vi "UHR-Fleezers Control (host) -TL FB Corrected Ronen semipassive - stepping.vi"(0 "Tab Control":T5(tab)=enum."Trap Control (RF)") -> ()   [LabVIEW 2013] (continued)
                      n1354 = To Double Precision Float(number=w2139) -> (double precision float=w2138:cluster{"Horizontal":dbl, "Vertical":dbl})
                      n1355 = Multiply(x=cluster{"Horizontal":dbl, "Vertical":dbl} {"Horizontal"=-1.0, "Vertical"=1.0}, y="Manipulation Scaling") -> (x*y=w2134:cluster{"Horizontal":dbl, "Vertical":dbl})
                      n1356 = local read "X RF Frequency Limits (MHz)"() -> (w2100:T17)
                      n1357 = Multiply(x=w2138, y=w2134) -> (x*y=w2136:cluster{"Horizontal":dbl, "Vertical":dbl})
                      n1358 = Unbundle By Name(w2136) -> ("Horizontal"=w2131:dbl, "Vertical"=w2135:dbl)
                      n1359 = Unbundle By Name(w2099) -> ("Maximum"=w2102:dbl, "Minimum"=w2101:dbl)
                      n1360 = Boolean To (0,1)(Boolean="Manip. X?") -> (0, 1=w2129:i16)
                      n1361 = Boolean To (0,1)(Boolean="Manip. Y?") -> (0, 1=w2126:i16)
                      n1362 = local read "BD 1 Frequency 2 (MHz)"() -> (w2116:dbl)
                      n1363 = Multiply(x=w2135, y=w2126) -> (x*y=w2128:dbl)
                      n1364 = Multiply(x=w2129, y=w2131) -> (x*y=w2132:dbl)
                      n1365 = local read "BD 2 Frequency 2 (MHz)"() -> (w2115:dbl)
                      n1366 = Unbundle By Name(w2100) -> ("Maximum"=w2104:dbl, "Minimum"=w2103:dbl)
                      n1367 = Add(x=w2113, y=w2128) -> (x+y=w2106:dbl)
                      n1368 = Add(x=w2114, y=w2132) -> (x+y=w2108:dbl)
                      n1369 = In Range and Coerce(upper limit=w2104, x=w2108, lower limit=w2103) -> (coerced(x)=w2107:dbl)  [unwired: 1 out]
                      n1370 = In Range and Coerce(upper limit=w2102, x=w2106, lower limit=w2101) -> (coerced(x)=w2105:dbl)  [unwired: 1 out]
                      n1371 = Subtract(x=w2107, y=w2116) -> (x-y=w2125:dbl)
                      n1372 = Subtract(x=w2105, y=w2115) -> (x-y=w2124:dbl)
                      n1373 = Square(x=w2125) -> (x^2=w2123:dbl)
                      n1374 = Square(x=w2124) -> (x^2=w2122:dbl)
                      n1375 = Add(x=w2123, y=w2122) -> (x+y=w2121:dbl)
                      n1376 = Square Root(x=w2121) -> (sqrt(x)=w2117:dbl)
                      n1377 = In Range and Coerce(upper limit="Limit Max (MHz)", x=w2117, lower limit="Limit Min (MHz)") -> (In Range?=w2110:bool)  [unwired: 1 out]
                      n1378 = Not(x="Limits Enable") -> (.not. x?=w2109:bool)
                      n1379 = Or(x=w2110, y=w2109) -> (x .or. y?=w2111:bool)
                      n1380 = case shown="True" w2111 {
                        tunnel: w2118 -> [_ w2151]
                        tunnel: w2117 -> [_ w2142]
                        tunnel: w2107 -> [_ w2149]
                        tunnel: w2116 -> [_ w2148]
                        tunnel: w2105 -> [_ w2147]
                        tunnel: w2115 -> [_ w2146]
                        tunnel: w2100 -> [_ w2144]
                        tunnel: w2099 -> [_ w2143]
                        frame False {
                        }
                        frame True {
                          n1381 = local read "BD 1 Frequency 3 (MHz)"() -> (w2150:dbl)
                          n1382 = local read "BD 2 Frequency 3 (MHz)"() -> (w2145:dbl)
                          n1383 = local write "Trap Delta (MHz)"(w2142) -> ()
                          n1384 = property on="Initial delta (MHz)" class="DigNum (strict)"("Val(Sgnl)"=w2142) -> ()  [unwired: 2 in, 2 out]
                          n1385 = call "set RF board frequency - interlace.vi"("Board 2 Frequency Limits"=w2143, "Board 1 Frequency Limits"=w2144, "FPGA VI Reference In"=w2151, "Board 2 Frequency 3 (MHz)"=w2145, "Board 1 Frequency 3 (MHz)"=w2150, "Board 2 Frequency 2 (MHz)"=w2146, "Board 2 Frequency 1 (MHz)"=w2147, "Board 1 Frequency 2 (MHz)"=w2148, "Board 1 Frequency 1  (MHz)"=w2149) -> ()  [unwired: 1 in, 2 out]
                          n1386 = local write "BD 2 Frequency 1 (MHz)"(w2147) -> ()
                          n1387 = local write "BD 1 Frequency 1 (MHz)"(w2149) -> ()
                        }
                      }
                    }
                    frame True {
                    }
                  }
                }
                event Mouse Up {
                  n1388 = event-data() -> ("Button"=w2152:u16)  [unwired: 8 out]
                  n1389 = case shown="3" w2152 {
                    tunnel: [FALSE TRUE] -> w2153
                    frame 0, Default {
                    }
                    frame 3 {
                      n1390 = local write "Manipulating Trap"(FALSE ("Manipulating Trap")) -> ()
                    }
                  }
                }
              }
            }
          }
        }
      }
      event Mouse Move {
        n1391 = event-data() -> ()  [unwired: 6 out]
      }
    }
    n1392 = local read "Stop All"() -> (w1974:bool)
    n1393 = node-c288() -> ()  [unwired: 2 out]
  }
  n1394 = node-c288(w34) -> ()  [unwired: 1 out]
  n1395 = node-c288(w88) -> ()  [unwired: 1 out]
  n1396 = node-c288(w95) -> ()  [unwired: 1 out]
  n1397 = node-c288(i64 1 ("Period"), 1 ("Processor")) -> (w182:T25)  [unwired: 2 out]
  n1398 = timed-loop "Acquire Data" {
    tunnel: w44 -> [w2440]
    tunnel: w60 -> [w2439]
    tunnel: [w2470] -> w53
    tunnel: [w2464] -> w52
    timing: w182 -> [_]
    timing-out: [_] -> w181
    tunnel: w79 -> [w2276]
    stop <- "Stop All" stop-if-true
    (unwired) u32 0 ("Number of Elements")
    w2263 = "NI_ChannelName" ("name")
    n1399 = node-c288() -> ()  [unwired: 2 out]
    n1400 = First Call?() -> (First Call?: T/F=w2229:bool)
    n1401 = Or(x="Reset", y=w2229) -> (x .or. y?=w2230:bool)
    n1402 = local read "MCL Tracking"() -> (w2167:bool)
    n1403 = case "Reset data stream" shown="True" w2230 {
      tunnel: w2440 -> [w2582 w2590]
      tunnel: w2439 -> [w2581 w2589]
      tunnel: [w2582 w2584] -> w2165
      tunnel: [w2581 w2583] -> w2435
      frame False {
      }
      frame True {
        w2587 = TRUE ("AI to FIFO")
        n1404 = local write "Overflow (data lost)"(FALSE ("Overflow (data lost)")) -> ()
        n1405 = call "reset FPGA DMA.vi"("error in"=w2589, "FPGA VI Reference In"=w2590) -> ("error out"=w2585:errorcluster, "FPGA VI Reference Out"=w2586:T20)
        n1406 = xnode "Read/Write Control"("FPGA VI Reference In"=w2586, "error in"=w2585, "AI to FIFO"=w2587, "APD to FIFO"=w2587) -> ("FPGA VI Reference Out"=w2584:T20, "error out"=w2583:errorcluster)
      }
    }
    n1407 = Or(x="Start AOD Scan", y="Trap Raster Scan") -> (x .or. y?=w2391:bool)
    n1408 = case "Start AOM raster scan" shown="True" w2391 {
      tunnel: w2165 -> [w3319 w3329]
      tunnel: w2435 -> [w3318 w3328]
      tunnel: [w3319 w3322] -> w2164
      tunnel: [w3318 w3321] -> w2434
      frame False {
      }
      frame True {
        n1409 = case shown="True" "Restart DMA? (AOD)" {
          tunnel: [w3367 w3369] -> w3323
          tunnel: [w3366 w3368] -> w3324
          tunnel: w3329 -> [w3367 w3371]
          tunnel: w3328 -> [w3366 w3370]
          frame False {
          }
          frame True {
            n1410 = local write "Overflow (data lost)"(FALSE ("Overflow (data lost)")) -> ()
            n1411 = call "reset FPGA DMA.vi"("error in"=w3370, "FPGA VI Reference In"=w3371) -> ("error out"=w3368:errorcluster, "FPGA VI Reference Out"=w3369:T20)
          }
        }
        n1412 = local write "Trap Raster Scan"(FALSE ("Trap Raster Scan")) -> ()
        n1413 = case shown="True" "Move MCL Also?" {
          tunnel: w3324 -> [w3332 w3361]
          tunnel: w3323 -> [w3333 w3362]
          tunnel: [w3331 w3365] -> w3322
          tunnel: [w3330 w3364] -> w3321
          frame False {
            w3334 = TRUE ("AI to FIFO")
            n1414 = xnode "Read/Write Control"("FPGA VI Reference In"=w3333, "error in"=w3332, "AI to FIFO"=w3334, "APD to FIFO"=w3334, "Start scan"=w3334) -> ("FPGA VI Reference Out"=w3331:T20, "error out"=w3330:errorcluster)
          }
          frame True {
            w3358 = FALSE ("1D or 2D Scan?")
            w3363 = TRUE ("AI to FIFO")
            # "Count for MCL loop"
            # "N total cycles"
            # "N steps"
            # "V_int"
            n1415 = local read "Scan Range (nm)"() -> (w3340:dbl)
            n1416 = local read "Number of F/B Scans (AOD)"() -> (w3357:u16)
            n1417 = Sign(1:w3340) -> (0:w3339:dbl)
            n1418 = Compound Arithmetic op=MULTIPLY(w3340, "MCL Step Position Ratio", "MCL/AOM Scale Tweak") -> (w3344:dbl)
            n1419 = Negate(x=w3339) -> (-x=w3336:dbl)
            n1420 = Multiply(x=w3336, y="MCL Step Increment (V_int)") -> (x*y=w3338:dbl)
            n1421 = Divide(x=w3344, y="MCL X Cal (nm/V)") -> (x/y=w3350:dbl)
            n1422 = Multiply(x=32767.0 ("y"), y=w3350) -> (x*y=w3356:dbl)
            n1423 = local read "Total Counts (ticks)"() -> (w3341:u32)
            n1424 = local read "Cycles/step (AOD)"() -> (w3352:u64)
            n1425 = local read "Scan steps (AOD)"() -> (w3353:u64)
            n1426 = Divide(x=w3356, y=10.0) -> (x/y=w3349:dbl)
            n1427 = Divide(x=w3349, y="MCL Step Increment (V_int)") -> (x/y=w3347:dbl)
            n1428 = Absolute Value(x=w3347) -> (abs(x)=w3335:dbl)
            n1429 = Compound Arithmetic op=MULTIPLY(w3353, w3352, w3341) -> (w3348:u64)
            n1430 = local write "wait to reset values"(w3363) -> ()
            n1431 = local write "MCL Scanning"(w3363) -> ()
            n1432 = Divide(x=w3348, y=w3335) -> (x/y=w3345:dbl)
            "MCL Count" <- w3345
            n1433 = xnode "Read/Write Control"("FPGA VI Reference In"=w3362, "error in"=w3361, "Scan steps (MCL)"=w3335, "Number of scans (MCL)"=w3357, "Cycles per step (MCL)"=u64 1, "Scan freq.  increment (MCL)"=w3338, "1D or 2D Scan?"=w3358, "MCL Scan Axis"=w3358, "Cont. Scan (MCL)"=w3358, "MCL count"=w3345) -> ("FPGA VI Reference Out"=w3360:T20, "error out"=w3359:errorcluster)
            n1434 = xnode "Read/Write Control"("FPGA VI Reference In"=w3360, "error in"=w3359, "AI to FIFO"=w3363, "APD to FIFO"=w3363, "Start scan"=w3363, "Start scan (MCL)"=w3363) -> ("FPGA VI Reference Out"=w3365:T20, "error out"=w3364:errorcluster)
          }
        }
        "Raster Scanning..." <- TRUE ("Scanning...")
      }
    }
    n1435 = And(x="Save scans", y=w2391) -> (x .and. y?=w2433:bool)
    n1436 = Compound Arithmetic op=OR("Start MCL Scan", "Confocal Image", "Confocal Linescan") -> (w2389:bool)
    n1437 = And(x="Save Data (MCL)", y=w2389) -> (x .and. y?=w2432:bool)
    n1438 = case "Start MCL raster scan" shown="True" w2389 {
      tunnel: w2164 -> [w2873 w2888]
      tunnel: w2434 -> [w2872 w2887]
      tunnel: [w2873 w2883] -> w2199
      tunnel: [w2872 w2882] -> w2198
      tunnel: [FALSE w2881] -> w2418
      tunnel: "Start MCL Scan" -> [_ w2876]
      tunnel: "Confocal Image" -> [_ w2875]
      tunnel: "Confocal Linescan" -> [_ _]
      frame False {
      }
      frame True {
        w2881 = TRUE
        n1439 = case shown="True" "Restart DMA? (MCL)" {
          tunnel: [w2933 w2935] -> w2886
          tunnel: [w2932 w2934] -> w2885
          tunnel: w2888 -> [w2933 w2938]
          tunnel: w2887 -> [w2932 w2937]
          frame False {
          }
          frame True {
            n1440 = call "reset FPGA DMA.vi"("error in"=w2937, "FPGA VI Reference In"=w2938) -> ("error out"=w2934:errorcluster, "FPGA VI Reference Out"=w2935:T20)
            n1441 = local write "Overflow (data lost)"(FALSE ("Overflow (data lost)")) -> ()
          }
        }
        n1442 = case shown="False" w2876 {
          selector: w2876 -> [_ w2892]
          tunnel: w2875 -> [w2891 _]
          tunnel: [w2891 w2892] -> w2874
          frame False {
            n1443 = property on="2D or 1D Scan" class="Bool (strict)"("Val(Sgnl)"=w2891) -> ()  [unwired: 2 in, 2 out]
            n1444 = property on="Confocal Image" class="Bool (strict)"("Value"=FALSE ("Start Confocal Map")) -> ()  [unwired: 2 in, 2 out]
          }
          frame True {
          }
        }
        n1445 = local write "MCL Scanning"(w2881) -> ()
        n1446 = local read "AO1"() -> (w2878:dbl)
        n1447 = local read "AO2"() -> (w2877:dbl)
        n1448 = case shown="True" "Center Scan" {
          tunnel: w2886 -> [w2899 w2931]
          tunnel: w2885 -> [w2898 w2930]
          tunnel: [w2897 w2929] -> w2883
          tunnel: [w2896 w2928] -> w2882
          tunnel: [w2894 w2915] -> w2880
          tunnel: [w2893 w2914] -> w2879
          tunnel: w2878 -> [w2894 w2920]
          tunnel: w2877 -> [w2893 w2923]
          tunnel: w2874 -> [_ _]
          frame False {
            w2895 = TRUE ("AI to FIFO")
            n1449 = xnode "Read/Write Control"("FPGA VI Reference In"=w2899, "error in"=w2898, "AI to FIFO"=w2895, "APD to FIFO"=w2895, "Start scan (MCL)"=w2895) -> ("FPGA VI Reference Out"=w2897:T20, "error out"=w2896:errorcluster)
          }
          frame True {
            w2927 = TRUE ("AI to FIFO")
            n1450 = local read "Scan steps (MCL)"() -> (w2906:u64)
            n1451 = local read "Scan lines (y)"() -> (w2902:u64)
            n1452 = local read "Fast Scan Dir"() -> (w2913:bool)
            n1453 = local read "Actual MCL Inc (V)"() -> (w2903:dbl)
            n1454 = Decrement(x=w2902) -> (x-1=w2901:u64)
            n1455 = Decrement(x=w2906) -> (x-1=w2905:u64)
            n1456 = Multiply(x=w2903, y=w2901) -> (x*y=w2900:dbl)
            n1457 = Divide(x=w2900, y=2.0) -> (x/y=w2910:dbl)
            n1458 = Multiply(x=w2903, y=w2905) -> (x*y=w2904:dbl)
            n1459 = Divide(x=w2904, y=2.0) -> (x/y=w2909:dbl)
            n1460 = Select(t=w2909, s=w2913, f=w2910) -> (s? t:f=w2908:dbl)
            n1461 = Select(t=w2910, s=w2913, f=w2909) -> (s? t:f=w2912:dbl)
            n1462 = Subtract(x=w2920, y=w2912) -> (x-y=w2911:dbl)
            n1463 = Subtract(x=w2923, y=w2908) -> (x-y=w2907:dbl)
            n1464 = local read "2D or 1D Scan"() -> (w2925:bool)
            n1465 = Not(x=w2913) -> (.not. x?=w2919:bool)
            n1466 = Not(x=w2925) -> (.not. x?=w2921:bool)
            n1467 = And(x=w2913, y=w2921) -> (x .and. y?=w2922:bool)
            n1468 = And(x=w2921, y=w2919) -> (x .and. y?=w2924:bool)
            n1469 = Select(t=w2923, s=w2924, f=w2907) -> (s? t:f=w2914:dbl)
            n1470 = Select(t=w2920, s=w2922, f=w2911) -> (s? t:f=w2915:dbl)
            n1471 = call "Volt to I16.vi"("Voltage In"=w2915) -> ("I16 Voltage Out"=w2918:i16)
            n1472 = call "Volt to I16.vi"("Voltage In"=w2914) -> ("I16 Voltage Out"=w2917:i16)
            n1473 = xnode "Read/Write Control"("FPGA VI Reference In"=w2931, "error in"=w2930, "AI to FIFO"=w2927, "APD to FIFO"=w2927, "Start scan (MCL)"=w2927, "AO1"=w2918, "AO2"=w2917) -> ("FPGA VI Reference Out"=w2929:T20, "error out"=w2928:errorcluster)
          }
        }
        "Initial Y" <- w2880
        "Initial X" <- w2879
        "wait to reset values" <- w2881
      }
    }
    n1474 = local read "Trap Pos Elements/DMA read"() -> (w2272:u32)
    n1475 = local read "Trap AI Elements/DMA read"() -> (w2197:u32)
    n1476 = local read "APD Elements/DMA read"() -> (w2315:u32)
    n1477 = local read "Trap AI FIFO Depth"() -> (w2480:u32)
    n1478 = xnode "Invoke Method"("FPGA VI Reference In"=w2199, "error in"=w2198, "Number of Elements"=w2272, "Timeout (ms)"=-1) -> ("Data"=w2236:u16[], "Elements Remaining"=→"Trap Pos FIFO El Remaining":u32)  [unwired: 2 out]
    n1479 = xnode "Invoke Method"("FPGA VI Reference In"=w2199, "error in"=w2198, "Number of Elements"=w2197, "Timeout (ms)"=-1 ("Timeout")) -> ("FPGA VI Reference Out"=w2168:T20, "error out"=w2200:errorcluster, "Data"=w2196:i16[], "Elements Remaining"=w2201:u32)
    "Trap AI FIFO El. Rem." <- w2201
    n1480 = xnode "Get APD Data"("FPGA VI Reference In"=w2199, "error in"=w2198, "Number of Elements"=w2315, "Timeout (ms)"=-1) -> ("Data"=w2314:u32[], "Elements Remaining"=→"APD FIFO Elements Remaining":u32)  [unwired: 2 out]
    n1481 = Subtract(x=w2480, y=w2197) -> (x-y=w2479:u32)
    n1482 = Decimate 1D Array(w2236) -> (w2233:u16[], w2235:u16[], w2234:u16[])
    n1483 = Divide(x=w2201, y=w2479) -> (x/y=w2478:dbl)
    "Buffer Status" <- w2478
    n1484 = To Unsigned Long Integer(number=w2233) -> (unsigned 32bit integer=w2232:u32[])
    n1485 = Join Numbers(hi=w2235, lo=w2234) -> ((hi.lo)=w2231:u32[])
    n1486 = Equal?(x=w2478, y=1.0) -> (x = y?=w2476:bool)
    n1487 = Join Numbers(hi=w2232, lo=w2231) -> ((hi.lo)=w2225:u64[])
    n1488 = call "IR AOM word to freq - vec.vi"("Frequency Word In (double vec)"=w2225) -> ("Frequency Out"=w2271:dbl[])
    n1489 = case "Alert buffer overflow" shown="False" w2476 {
      frame False {
      }
      frame True {
        n1490 = call <vilib>:"Beep.vi"() -> ()  [unwired: 3 in, 9 out]
        "Overflow (data lost)" <- TRUE ("Overflow (data lost)")
      }
    }
    n1491 = Decimate 1D Array(w2271) -> (w2270:dbl[], w2269:dbl[])
    n1492 = Array Size(array=w2196) -> (size(s)=→"Waveform Chart":i32)
    n1493 = Build Array(w2270, w2269) -> (w2268:dbl[][])
    n1494 = local read "Trap Sets"() -> (w2351:u32)
    n1495 = case "Deinterlace trap data, average down PSD" shown="2" w2351 {
      tunnel: w2196 -> [w2968 w3033]
      tunnel: [w2965 w3030] -> w2344
      tunnel: [w2968 w3032] -> w2228
      tunnel: "Detector Type" -> [w2967 w3028]
      tunnel: [w2966 w3031] -> w2343
      tunnel: [w2964 w3029] -> w2451
      frame 1, Default {
        n1496 = Divide(x=w2968, y=3276.7) -> (x/y=w2969:dbl[])
        n1497 = Decimate 1D Array(w2969) -> (w2978:dbl[], w2977:dbl[], w2976:dbl[], w2975:dbl[], w2974:dbl[], w2973:dbl[], w2972:dbl[], w2971:dbl[])
        n1498 = case shown="\"IR-QPD + PSD + FB-QPD position\"" w2967 {
          tunnel: w2978 -> [w3002 w3027]
          tunnel: w2977 -> [w3001 w3026]
          tunnel: w2976 -> [w2986 w3004]
          tunnel: w2975 -> [w2987 w3014]
          tunnel: w2974 -> [w3000 w3025]
          tunnel: w2973 -> [w2999 w3024]
          tunnel: w2972 -> [w2983 w3005]
          tunnel: w2971 -> [w2982 w3003]
          tunnel: [w2981 w3011] -> w2966
          tunnel: [w2980 w3010] -> w2965
          tunnel: [w2979 w3009] -> w2964
          frame "IR-QPD + PSD + FB-QPD", Default {
            w2979 = 0  # Channel pattern
            n1499 = Divide(x=w3002, y=w2987) -> (x/y=w2989:dbl[])
            n1500 = Divide(x=w3001, y=w2987) -> (x/y=w2988:dbl[])
            n1501 = Divide(x=w3000, y=w2983) -> (x/y=w2985:dbl[])
            n1502 = Divide(x=w2999, y=w2982) -> (x/y=w2984:dbl[])
            n1503 = Build Array(w2989, w2988, w2987, w2986, w2985, w2984, w2983, w2982) -> (w2980:dbl[][])
            n1504 = Bundle("T1 Y", "T1 X", "T1 Sum", "FB Sum", "PSD Y", "PSD X", "PSD Y Sum", "PSD X Sum") -> (w2998:T42)  [unwired: 1 out]
            n1505 = Cluster To Array(cluster=w2998) -> (array=w2981:string[])
          }
          frame "IR-QPD + PSD + FB-QPD position" {
            w3009 = 3  # Channel pattern
            n1506 = Negate(x=w3005) -> (-x=w3006:dbl[])
            n1507 = Divide(x=w3027, y=w3014) -> (x/y=w3016:dbl[])
            n1508 = Divide(x=w3026, y=w3014) -> (x/y=w3015:dbl[])
            n1509 = Divide(x=w3025, y=w3005) -> (x/y=w3013:dbl[])
            n1510 = Divide(x=w3024, y=w3006) -> (x/y=w3012:dbl[])
            n1511 = Build Array(w3016, w3015, w3014, w3003, w3004, w3013, w3012, w3005) -> (w3010:dbl[][])
            n1512 = Bundle("T1 Y", "T1 X", "T1 Sum", "FB X", "FB Sum", "PSD Y", "PSD X", "PSD Y Sum") -> (w3023:T42)  [unwired: 1 out]
            n1513 = Cluster To Array(cluster=w3023) -> (array=w3011:string[])
          }
        }
      }
      frame 2 {
        n1514 = case shown="\"UCB Fleezers 052511\"" w3028 {
          tunnel: w3033 -> [w3095 w3162 w3190 w3297]
          tunnel: [w3034 w3154 w3185 w3228] -> w3032
          tunnel: [w3061 w3145 w3187 w3275] -> w3031
          tunnel: [w3060 w3109 w3164 w3242] -> w3030
          tunnel: [w3054 w3144 w3227 w3273] -> w3029
          frame "IR-QPD + PSD + FB-QPD", Default {
            w3054 = 1  # Channel pattern
            # "time average x2 the 4th signal and the 4 psd signals (detection laser)"
            # "deinterlace 3 signals from qpd"
            n1515 = Decimate 1D Array(w3095) -> (w3094:i16[], w3093:i16[], w3059:i16[], w3092:i16[], w3082:i16[], w3080:i16[], w3079:i16[], w3077:i16[])
            n1516 = call "downsample 1D array - double.vi"("Ave N"=2.0, "Array In"=w3082) -> ("Array Out"=w3081:dbl[])  [unwired: 1 out]
            n1517 = call "downsample 1D array - double.vi"("Ave N"=2.0, "Array In"=w3077) -> ("Array Out"=w3076:dbl[])  [unwired: 1 out]
            n1518 = call "downsample 1D array - double.vi"("Ave N"=2.0, "Array In"=w3079) -> ("Array Out"=w3078:dbl[])  [unwired: 1 out]
            n1519 = call "downsample 1D array - double.vi"("Ave N"=2.0, "Array In"=w3080) -> ("Array Out"=w3062:dbl[])  [unwired: 1 out]
            n1520 = Decimate 1D Array(w3094) -> (w3091:i16[], w3063:i16[])
            n1521 = Decimate 1D Array(w3093) -> (w3090:i16[], w3088:i16[])
            n1522 = Decimate 1D Array(w3092) -> (w3089:i16[], w3087:i16[])
            n1523 = Decimate 1D Array(w3059) -> (w3058:i16[], w3057:i16[])
            n1524 = Interleave 1D Arrays(w3091, w3090, w3089, w3063, w3088, w3087, w3058, w3057, w3081, w3062, w3078, w3076) -> (w3075:dbl[])
            n1525 = To Word Integer(number=w3075) -> (16bit integer=w3034:i16[])
            n1526 = Divide(x=w3075, y=3276.7) -> (x/y=w3074:dbl[])
            n1527 = Decimate 1D Array(w3074) -> (w3073:dbl[], w3072:dbl[], w3071:dbl[], w3070:dbl[], w3069:dbl[], w3068:dbl[], w3056:dbl[], w3055:dbl[], w3067:dbl[], w3066:dbl[], w3065:dbl[], w3064:dbl[])
            n1528 = Divide(x=w3073, y=w3071) -> (x/y=w3041:dbl[])
            n1529 = Divide(x=w3072, y=w3071) -> (x/y=w3040:dbl[])
            n1530 = Divide(x=w3070, y=w3068) -> (x/y=w3039:dbl[])
            n1531 = Divide(x=w3069, y=w3068) -> (x/y=w3038:dbl[])
            n1532 = Divide(x=w3067, y=w3065) -> (x/y=w3037:dbl[])
            n1533 = Divide(x=w3066, y=w3064) -> (x/y=w3036:dbl[])
            n1534 = Bundle("T1 Y", "T1 X", "T1 Sum", "T2 Y", "T2 X", "T2 Sum", "T1 FB Sum", "T2 FB Sum", "PSD Y", "PSD X", "PSD Y Sum", "PSD X Sum") -> (w3042:T43)  [unwired: 1 out]
            n1535 = Build Array(w3041, w3040, w3071, w3039, w3038, w3068, w3056, w3055, w3037, w3036, w3065, w3064) -> (w3060:dbl[][])
            n1536 = Cluster To Array(cluster=w3042) -> (array=w3061:string[])
          }
          frame "IR-QPD + PSD + FB-QPD X position" {
            w3144 = 2  # Channel pattern
            # "convert\nADC numbers\nto volts"
            # "time average x2 the 3 psd signals (detection laser)"
            # "deinterlace 3 signals from qpds"
            n1537 = Decimate 1D Array(w3162) -> (w3161:i16[], w3160:i16[], w3097:i16[], w3098:i16[], w3107:i16[], w3104:i16[], w3101:i16[], w3132:i16[])
            n1538 = Decimate 1D Array(w3161) -> (w3159:i16[], w3146:i16[])
            n1539 = call "downsample 1D array - I16.vi"("Ave N"=2.0, "Array In"=w3107) -> ("Array Out"=w3105:i16[])  [unwired: 1 in]
            n1540 = call "downsample 1D array - I16.vi"("Ave N"=2.0, "Array In"=w3104) -> ("Array Out"=w3102:i16[])  [unwired: 1 in]
            n1541 = Decimate 1D Array(w3160) -> (w3158:i16[], w3156:i16[])
            n1542 = Decimate 1D Array(w3098) -> (w3157:i16[], w3155:i16[])
            n1543 = Decimate 1D Array(w3132) -> (w3131:i16[], w3129:i16[])
            n1544 = Decimate 1D Array(w3097) -> (w3130:i16[], w3128:i16[])
            n1545 = call "downsample 1D array - I16.vi"("Ave N"=2.0, "Array In"=w3101) -> ("Array Out"=w3099:i16[])  [unwired: 1 in]
            n1546 = Interleave 1D Arrays(w3159, w3158, w3157, w3146, w3156, w3155, w3131, w3130, w3129, w3128, w3105, w3102, w3099) -> (w3154:i16[])
            n1547 = Divide(x=w3154, y=3276.7) -> (x/y=w3153:dbl[])
            n1548 = Decimate 1D Array(w3153) -> (w3152:dbl[], w3151:dbl[], w3150:dbl[], w3149:dbl[], w3148:dbl[], w3147:dbl[], w3120:dbl[], w3118:dbl[], w3117:dbl[], w3115:dbl[], w3114:dbl[], w3113:dbl[], w3110:dbl[])
            n1549 = Divide(x=w3152, y=w3150) -> (x/y=w3136:dbl[])
            n1550 = Divide(x=w3151, y=w3150) -> (x/y=w3135:dbl[])
            n1551 = Divide(x=w3149, y=w3147) -> (x/y=w3134:dbl[])
            n1552 = Divide(x=w3148, y=w3147) -> (x/y=w3133:dbl[])
            n1553 = Divide(x=w3120, y=w3118) -> (x/y=w3119:dbl[])
            n1554 = Divide(x=w3117, y=w3115) -> (x/y=w3116:dbl[])
            n1555 = Divide(x=w3114, y=w3110) -> (x/y=w3112:dbl[])
            n1556 = Negate(x=w3110) -> (-x=w3108:dbl[])
            n1557 = Divide(x=w3113, y=w3108) -> (x/y=w3111:dbl[])
            n1558 = Bundle("T1 Y", "T1 X", "T1 Sum", "T2 Y", "T2 X", "T2 Sum", "T1 FB X", "T1 FB Sum", "T2 FB X", "T2 FB Sum", "PSD Y", "PSD X", "PSD Y Sum") -> (w3137:T44)  [unwired: 1 out]
            n1559 = Build Array(w3136, w3135, w3150, w3134, w3133, w3147, w3119, w3118, w3116, w3115, w3112, w3111, w3110) -> (w3109:dbl[][])
            n1560 = Cluster To Array(cluster=w3137) -> (array=w3145:string[])
          }
          frame "UCB Fleezers 052511" {
            w3227 = 2  # Channel pattern
            n1561 = Decimate 1D Array(w3190) -> (w3225:i16[], w3224:i16[], w3189:i16[], w3188:i16[], w3182:i16[], w3179:i16[], w3178:i16[], w3177:i16[])
            n1562 = Decimate 1D Array(w3225) -> (w3223:i16[], w3208:i16[])
            n1563 = Decimate 1D Array(w3224) -> (w3222:i16[], w3220:i16[])
            n1564 = Decimate 1D Array(w3189) -> (w3221:i16[], w3219:i16[])
            n1565 = Decimate 1D Array(w3188) -> (w3184:i16[], w3183:i16[])
            n1566 = Decimate 1D Array(w3182) -> (w3181:i16[], w3180:i16[])
            n1567 = call "downsample 1D array - I16.vi"("Ave N"=2.0, "Array In"=w3179) -> ("Array Out"=w3176:i16[])  [unwired: 1 in]
            n1568 = call "downsample 1D array - I16.vi"("Ave N"=2.0, "Array In"=w3178) -> ("Array Out"=w3175:i16[])  [unwired: 1 in]
            n1569 = call "downsample 1D array - I16.vi"("Ave N"=2.0, "Array In"=w3177) -> ("Array Out"=w3174:i16[])  [unwired: 1 in]
            n1570 = Interleave 1D Arrays(w3223, w3222, w3221, w3208, w3220, w3219, w3184, w3181, w3183, w3180, w3176, w3175, w3174) -> (w3185:i16[])
            n1571 = Divide(x=w3185, y=3276.7) -> (x/y=w3215:dbl[])
            n1572 = Decimate 1D Array(w3215) -> (w3214:dbl[], w3213:dbl[], w3212:dbl[], w3211:dbl[], w3210:dbl[], w3209:dbl[], w3173:dbl[], w3171:dbl[], w3170:dbl[], w3168:dbl[], w3167:dbl[], w3166:dbl[], w3165:dbl[])
            n1573 = Divide(x=w3214, y=w3212) -> (x/y=w3195:dbl[])
            n1574 = Divide(x=w3213, y=w3212) -> (x/y=w3194:dbl[])
            n1575 = Divide(x=w3211, y=w3209) -> (x/y=w3193:dbl[])
            n1576 = Divide(x=w3210, y=w3209) -> (x/y=w3192:dbl[])
            n1577 = Divide(x=w3173, y=w3171) -> (x/y=w3172:dbl[])
            n1578 = Divide(x=w3170, y=w3168) -> (x/y=w3169:dbl[])
            n1579 = Bundle("T1 Y", "T1 X", "T1 Sum", "T2 Y", "T2 X", "T2 Sum", "T1 FB X", "T2 FB Sum", "T2 FB X", "T2 FB Sum", "PSD Y", "PSD X", "PSD Sum") -> (w3196:T44)  [unwired: 1 out]
            n1580 = Build Array(w3195, w3194, w3212, w3193, w3192, w3209, w3172, w3171, w3169, w3168, w3167, w3166, w3165) -> (w3164:dbl[][])
            n1581 = Cluster To Array(cluster=w3196) -> (array=w3187:string[])
          }
          frame "IR-QPD + PSD + FB-QPD XY positions" {
            w3273 = 4  # Channel pattern
            # "time average x2 the 3 psd signals (detection laser)"
            # "deinterlace 3 signals from qpds"
            n1582 = Decimate 1D Array(w3297) -> (w3296:i16[], w3295:i16[], w3274:i16[], w3294:i16[], w3240:i16[], w3286:i16[], w3285:i16[], w3262:i16[])
            n1583 = Decimate 1D Array "QPD Y"(w3296) -> (w3293:i16[], w3276:i16[])
            n1584 = call "downsample 1D array - double.vi"("Ave N"=2.0, "Array In"=w3286) -> ("Array Out"=w3261:dbl[])  [unwired: 1 out]
            n1585 = call "downsample 1D array - double.vi"("Ave N"=2.0, "Array In"=w3285) -> ("Array Out"=w3260:dbl[])  [unwired: 1 out]
            n1586 = Decimate 1D Array "Feedback Sum"(w3274) -> (w3258:i16[], w3256:i16[])
            n1587 = Decimate 1D Array "Feedback Y"(w3240) -> (w3239:i16[], w3238:i16[])
            n1588 = Decimate 1D Array "Feedback X"(w3262) -> (w3259:i16[], w3257:i16[])
            n1589 = Decimate 1D Array "QPD Sum"(w3294) -> (w3291:i16[], w3289:i16[])
            n1590 = Decimate 1D Array "QPD X"(w3295) -> (w3292:i16[], w3290:i16[])
            n1591 = Interleave 1D Arrays(w3293, w3292, w3291, w3276, w3290, w3289, w3239, w3259, w3258, w3238, w3257, w3256, w3261, w3260) -> (w3284:dbl[])
            n1592 = To Word Integer(number=w3284) -> (16bit integer=w3228:i16[])
            n1593 = Divide(x=w3284, y=3276.7) -> (x/y=w3283:dbl[])
            n1594 = Decimate 1D Array(w3283) -> (w3282:dbl[], w3281:dbl[], w3280:dbl[], w3279:dbl[], w3278:dbl[], w3277:dbl[], w3235:dbl[], w3249:dbl[], w3233:dbl[], w3234:dbl[], w3247:dbl[], w3231:dbl[], w3245:dbl[], w3243:dbl[])
            n1595 = Divide(x=w3282, y=w3280) -> (x/y=w3266:dbl[])
            n1596 = Divide(x=w3281, y=w3280) -> (x/y=w3265:dbl[])
            n1597 = Divide(x=w3279, y=w3277) -> (x/y=w3264:dbl[])
            n1598 = Divide(x=w3278, y=w3277) -> (x/y=w3263:dbl[])
            n1599 = Divide(x=w3235, y=w3233) -> (x/y=w3232:dbl[])
            n1600 = Divide(x=w3249, y=w3233) -> (x/y=w3248:dbl[])
            n1601 = Divide(x=w3234, y=w3231) -> (x/y=w3230:dbl[])
            n1602 = Divide(x=w3247, y=w3231) -> (x/y=w3246:dbl[])
            n1603 = Negate(x=w3243) -> (-x=w3241:dbl[])
            n1604 = Divide(x=w3245, y=w3241) -> (x/y=w3244:dbl[])
            n1605 = Bundle("T1 Y", "T1 X", "T1 Sum", "T2 Y", "T2 X", "T2 Sum", "T1 FB Y", "T1 FB X", "T1 FB Sum", "T2 FB Y", "T2 FB X", "T2 FB Sum", "PSD X", "PSD Y Sum") -> (w3229:T45)  [unwired: 1 out]
            n1606 = Build Array(w3266, w3265, w3280, w3264, w3263, w3277, w3232, w3248, w3233, w3230, w3246, w3231, w3244, w3243) -> (w3242:dbl[][])
            n1607 = Cluster To Array(cluster=w3229) -> (array=w3275:string[])
          }
        }
      }
    }
    "AI labels" <- w2343
    n1608 = xnode "Read/Write Control"("FPGA VI Reference In"=w2168) -> ("FPGA VI Reference Out"=w2161:T20, "BD1 Frequency Out 1"=w2182:u64)  [unwired: 1 in, 1 out]
    n1609 = local read "BD 1 Frequency 2 (MHz)"() -> (w2173:dbl)
    n1610 = To Double Precision Float(number=w2182) -> (double precision float=w2179:dbl)
    n1611 = Multiply(x=49125000.0, y=6.0) -> (x*y=w2178:dbl)
    n1612 = Multiply(x=w2179, y=w2178) -> (x*y=w2176:dbl)
    n1613 = Scale By Power Of 2(n=-48, x=w2176) -> (x*2^n=w2175:dbl)
    n1614 = local read "Dynamic Force FB"() -> (w2172:bool)
    n1615 = local read "Trap Pos. FB ON"() -> (w2171:bool)
    n1616 = Divide(x=w2175, y=1000000.0) -> (x/y=w2166:dbl)
    n1617 = case shown="True" w2167 {
      tunnel: w2166 -> [_ w2557]
      tunnel: w2164 -> [_ w2544]
      frame False {
      }
      frame True {
        n1618 = local read "AOM X Cal (nm/MHz)"() -> (w2554:dbl)
        n1619 = local read "Zero T1 position"() -> (w2556:dbl)
        n1620 = Subtract(x=w2557, y=w2556) -> (x-y=w2555:dbl)
        n1621 = Multiply(x=w2555, y=w2554) -> (x*y=w2553:dbl)
        n1622 = local read "MCL X Cal (nm/V)"() -> (w2550:dbl)
        n1623 = Multiply(x=w2553, y="Tracking factor") -> (x*y=w2551:dbl)
        n1624 = local read "Zero MCL x position"() -> (w2549:dbl)
        n1625 = Divide(x=w2551, y=w2550) -> (x/y=w2548:dbl)
        n1626 = Add(x=w2549, y=w2548) -> (x+y=w2541:dbl)
        "Current MCL (V)" <- w2541
        n1627 = Multiply(x=w2541, y=32767.0) -> (x*y=w2545:dbl)
        n1628 = Divide(x=w2545, y=10.0) -> (x/y=w2542:dbl)
        n1629 = To Word Integer(number=w2542) -> (16bit integer=w2543:i16)
        n1630 = xnode "Read/Write Control"("FPGA VI Reference In"=w2544, "AO2"=w2543) -> ()  [unwired: 1 in, 2 out]
      }
    }
    n1631 = Subtract(x=w2173, y=w2166) -> (x-y=w2162:dbl)
    "Current deltaFreq" <- w2162
    n1632 = Compound Arithmetic op=AND(w2172, w2171, "Real time offset \ncorrection for setpoint") -> (w2169:bool)
    n1633 = case shown="True" w2169 {
      tunnel: w2162 -> [_ w2560]
      tunnel: w2161 -> [_ w2559]
      frame False {
      }
      frame True {
        n1634 = local read "T1 kappa_x (pN/nm)"() -> (w2568:dbl)
        n1635 = local read "T1 alpha_x (nm/V)"() -> (w2569:dbl)
        n1636 = local read "Negate offset difference"() -> (w2570:bool)
        n1637 = local read "Offset file step size"() -> (w2578:dbl)
        n1638 = Multiply(x="Target Force (pN)", y=2.0) -> (x*y=w2566:dbl)
        n1639 = local read "Setpoint offset\nCorrection values"() -> (w2575:dbl[])
        n1640 = Divide(x=w2560, y=w2578) -> (x/y=w2577:dbl)
        n1641 = Select(t=-1, s=w2570, f=1) -> (s? t:f=w2571:i32)
        n1642 = To Long Integer(number=w2577) -> (32bit integer=w2576:i32)
        n1643 = Multiply(x=w2569, y=w2568) -> (x*y=w2565:dbl)
        n1644 = Divide(x=w2566, y=w2565) -> (x/y=w2564:dbl)
        n1645 = Index Array(array=w2575, index=w2576) -> (element=w2574:dbl)
        n1646 = Multiply(x=w2571, y=w2574) -> (x*y=w2563:dbl)
        n1647 = Add(x=w2564, y=w2563) -> (x+y=w2562:dbl)
        n1648 = To Fixed-Point(number=w2562) -> (fixed-point=w2558:fxp<+/-,16,1>)  [unwired: 1 in]
        "Actual setpoint" <- w2558
        n1649 = xnode "Read/Write Control"("FPGA VI Reference In"=w2559, "Trap Pos. FB SP"=w2558) -> ()  [unwired: 1 in, 2 out]
      }
    }
    n1650 = case shown="False" "Take full offset data for display" {
      tunnel: [w2527 w2533] -> w2368
      tunnel: [w2526 w2532] -> w2366
      tunnel: w2162 -> [_ w2539]
      frame False {
        n1651 = Divide(x="T2 offset_x (mV)", y=1000.0) -> (x/y=w2526:dbl)
        n1652 = Divide(x="T1 offset_x (mV)", y=1000.0) -> (x/y=w2527:dbl)
      }
      frame True {
        n1653 = local read "Offset Values"() -> (w2540:T14)
        n1654 = local read "Offset file step size"() -> (w2538:dbl)
        n1655 = Unbundle By Name(w2540) -> ("Trap 1X offset"=w2535:dbl[], "Trap 2X offset"=w2534:dbl[])
        n1656 = Divide(x=w2539, y=w2538) -> (x/y=w2537:dbl)
        n1657 = To Long Integer(number=w2537) -> (32bit integer=w2536:i32)
        n1658 = Index Array(array=w2535, index=w2536) -> (element=w2533:dbl)
        n1659 = Index Array(array=w2534, index=w2536) -> (element=w2532:dbl)
      }
    }
    n1660 = Decimate 1D Array(w2314) -> (w2341:u32[], w2278:u32[])
    n1661 = local read "DMA Update Period (s)"() -> (w2352:dbl)
    n1662 = local read "BD 1 Frequency 2 (MHz)"() -> (w2220:dbl)
    n1663 = local read "BD 1 Frequency 1 (MHz)"() -> (w2221:dbl)
    n1664 = Build Array(w2341, w2278) -> (w2415:u32[][])
    n1665 = local read "Data Period (s)"() -> (w2327:dbl)
    n1666 = Decimate 1D Array(w2228) -> (w2251:i16[], w2250:i16[], w2248:i16[], w2247:i16[])  [unwired: 9 out]
    n1667 = To Double Precision Float(number=w2415) -> (double precision float=w2416:dbl[][])
    n1668 = local read "APD Integration Time (s)"() -> (w2291:dbl)
    n1669 = Divide(x=w2251, y=w2250) -> (x/y=w2252:dbl[])
    n1670 = Divide(x=w2248, y=w2247) -> (x/y=w2249:dbl[])
    n1671 = feedback #1(0.0) -> (w2265:dbl)
    n1672 = Add(x=w2352, y=w2265) -> (x+y=w2453:dbl)
    n1673 = feedback-in #1(w2453) -> ()
    n1674 = local read "AOM X Cal (nm/MHz)"() -> (w2218:dbl)
    n1675 = To Time Stamp(1:w2265) -> (0:w2264:timestamp)
    n1676 = Split 1D Array(array=w2252, index="N El. to Ave.") -> (second subarray=w2255:dbl[])  [unwired: 1 out]
    n1677 = Split 1D Array(array=w2249, index="N El. to Ave.") -> (second subarray=w2254:dbl[])  [unwired: 1 out]
    n1678 = local read "Trap X AI1 (DMA)"() -> (w2253:T13)
    n1679 = Multiply(x=w2327, y="Trap Disp. Downsample") -> (x*y=w2266:dbl)
    "Display Period (s)" <- w2266
    n1680 = Bundle("BD 1 Frequency 1 (MHz)"=w2221, "BD 1 Frequency 2 (MHz)"=w2220) -> (w2222:T46)  [unwired: 1 out]
    n1681 = for "Trap AI" {
      tunnel: [w2963] -> w2447 mode=indexing
      tunnel: w2264 -> [w2953]
      tunnel: "Trap Disp. Downsample" -> [w2961]
      tunnel: w2344 -> [w2959] mode=indexing
      tunnel: w2327 -> [w2958]
      tunnel: w2343 -> [w2957] mode=indexing
      tunnel: w2263 -> [w2956]
      tunnel: [w2955] -> w2302 mode=indexing
      tunnel: w2266 -> [w2954]
      n1682 = Bundle By Name("Y"=w2959, "dt"=w2958) -> (w2960:waveform(dbl))  [unwired: 1 out]
      n1683 = Set Waveform Attribute(5:w2957, 6:w2956, 7:w2960) -> (3:w2955:waveform(dbl))  [unwired: 1 in, 2 out]
      n1684 = call "downsample 1D array - double.vi"("Ave N"=w2961, "Array In"=w2959) -> ("Array Out"=w2962:dbl[])  [unwired: 1 out]
      n1685 = Bundle By Name(cluster=w2955, "t0"=w2953, "Y"=w2962, "dt"=w2954) -> (w2963:waveform(dbl))
    }
    n1686 = call-poly <vilib>:"Mean.vi"("X"=w2254) -> ("mean"=w2242:dbl)  [unwired: 1 out]
    n1687 = call-poly <vilib>:"Mean.vi"("X"=w2255) -> ("mean"=w2243:dbl)  [unwired: 1 out]
    n1688 = Cluster To Array(cluster=w2222) -> (array=w2219:dbl[])
    n1689 = Reciprocal(x=w2266) -> (1/x=→"Trap Disp. Freq. (Hz)":dbl)
    n1690 = local read "Data points/scans (MCL)"() -> (w2427:dbl)
    n1691 = To Fixed-Point(number=w2242) -> (fixed-point=w2240:fxp<+/-,16,1>)  [unwired: 1 in]
    n1692 = To Fixed-Point(number=w2243) -> (fixed-point=w2241:fxp<+/-,16,1>)  [unwired: 1 in]
    n1693 = Bundle("Trap 1 Pos.", "Trap 2 Pos.") -> (w2262:cluster{string, string})  [unwired: 1 out]
    n1694 = Bundle By Name(cluster=w2253, "Set 1"=w2241, "Set 2"=w2240) -> (→"Trap X AI1 (DMA)":T13)
    n1695 = Cluster To Array(cluster=w2262) -> (array=w2259:string[])
    n1696 = for "Trap Position" {
      tunnel: w2268 -> [w2603] mode=indexing
      tunnel: "Trap Disp. Downsample" -> [w2602]
      tunnel: w2266 -> [w2600]
      tunnel: w2264 -> [w2599]
      tunnel: w2263 -> [w2597]
      tunnel: w2259 -> [w2596] mode=indexing
      tunnel: [w2595] -> w2217 mode=indexing
      tunnel: w2219 -> [w2593] mode=indexing
      tunnel: w2218 -> [w2591]
      n1697 = call "downsample 1D array - double.vi"("Ave N"=w2602, "Array In"=w2603) -> ("Array Out"=w2601:dbl[])  [unwired: 1 out]
      n1698 = Subtract(x=w2601, y=w2593) -> (x-y=w2594:dbl[])
      n1699 = Multiply(x=w2591, y=w2594) -> (x*y=w2592:dbl[])
      n1700 = Bundle By Name("Y"=w2592, "dt"=w2600, "t0"=w2599) -> (w2598:waveform(dbl))  [unwired: 1 out]
      n1701 = Set Waveform Attribute(5:w2596, 6:w2597, 7:w2598) -> (3:w2595:waveform(dbl))  [unwired: 1 in, 2 out]
    }
    "Trap Positions" <- w2217
    n1702 = Bundle("APD 1", "APD 2") -> (w2446:cluster{string, string})  [unwired: 1 out]
    n1703 = Cluster To Array(cluster=w2446) -> (array=w2443:string[])
    n1704 = for "APD" {
      tunnel: w2416 -> [w2942] mode=indexing
      tunnel: w2291 -> [w2950]
      tunnel: [w2946] -> w2298 mode=indexing
      tunnel: "APD Disp. Scale" -> [w2947]
      tunnel: w2263 -> [w2945]
      tunnel: w2443 -> [w2944] mode=indexing
      tunnel: "APD Disp. Downsample" -> [w2940]
      tunnel: [w2943] -> w2442
      tunnel: w2264 -> [w2939]
      n1705 = call "integrate 1D array interval - double.vi"("Ave N"=w2940, "Array In"=w2942) -> ("Array Out"=w2941:dbl[])  [unwired: 1 out]
      n1706 = Multiply(x=w2950, y=w2940) -> (x*y=w2943:dbl)
      n1707 = Divide(x=w2941, y=w2947) -> (x/y=w2948:dbl[])
      n1708 = Bundle By Name("t0"=w2939, "Y"=w2948, "dt"=w2943) -> (w2949:waveform(dbl))  [unwired: 1 out]
      n1709 = Set Waveform Attribute(5:w2944, 6:w2945, 7:w2949) -> (3:w2946:waveform(dbl))  [unwired: 1 in, 2 out]
    }
    "APD Display Period (s)" <- w2442
    n1710 = Reciprocal(x=w2442) -> (1/x=→"APD Display Freq. (Hz)":dbl)
    n1711 = local read "Display Period (s)"() -> (w2326:dbl)
    n1712 = Increment(x=w2427) -> (x+1=w2428:dbl)
    n1713 = Index Array(array=w2217, index=0) -> (element=w2215:waveform(dbl))
    n1714 = To Double Precision Float(number=w2341) -> (double precision float=w2340:dbl[])
    n1715 = feedback #2(w2428) -> (w2431:dbl)
    n1716 = Select(t=0, s=w2418, f=w2431) -> (s? t:f=w2424:dbl)
    n1717 = Array Size(array=w2340) -> (size(s)=w2430:i32)
    n1718 = Add(x=w2430, y=w2424) -> (x+y=w2425:dbl)
    n1719 = Unbundle By Name(w2215) -> ("Y"=w2213:dbl[])
    n1720 = feedback #3(w2341) -> (w2414:u32[])
    n1721 = Build Array (concatenate)(w2414, w2341) -> (w2411:u32[])
    n1722 = feedback #4(w2278) -> (w2297:u32[])
    n1723 = Divide(x="Bead Sep. Int. Time (s)", y=w2326) -> (x/y=w2211:dbl)
    n1724 = Build Array (concatenate)(w2297, w2278) -> (w2296:u32[])
    n1725 = Greater?(x=w2425, y=w2427) -> (0:w2426:bool)
    n1726 = feedback #5(w2213) -> (w2214:dbl[])
    n1727 = Build Array (concatenate)(w2213, w2214) -> (w2212:dbl[])
    n1728 = Select(t=w2424, s=w2426, f=w2425) -> (s? t:f=w2423:dbl)
    n1729 = feedback-in #2(w2423) -> ()
    n1730 = Array Size(array=w2411) -> (size(s)=w2408:i32)
    n1731 = Array Size(array=w2341) -> (size(s)=w2410:i32)
    n1732 = local read "MCL Scanning"() -> (w2421:bool)
    n1733 = local read "APD Integration Time (s)"() -> (w2305:dbl)
    n1734 = Build Array (concatenate)(w2298, w2447) -> (w2300:waveform(dbl)[])
    "All Signals" <- w2300
    n1735 = Split 1D Array(array=w2212, index=w2211) -> (first subarray=w2205:dbl[])  [unwired: 1 out]
    n1736 = feedback-in #5(w2205) -> ()
    n1737 = Multiply(x=w2410, y="APD Ave N") -> (x*y=w2409:dbl)
    n1738 = Greater?(x=w2408, y=w2409) -> (0:w2412:bool)
    n1739 = Not(x=w2426) -> (.not. x?=w2420:bool)
    n1740 = To Double Precision Float(number=w2278) -> (double precision float=w2277:dbl[])
    n1741 = call-poly <vilib>:"Mean.vi"("X"=w2205) -> ("mean"=w2204:dbl)  [unwired: 1 out]
    "Mean T1 Position (nm)" <- w2204
    n1742 = Subtract(x=w2205, y=w2204) -> (x-y=w2210:dbl[])
    n1743 = Square(x=w2210) -> (x^2=w2209:dbl[])
    n1744 = And(x=w2420, y=w2421) -> (x .and. y?=w2422:bool)
    n1745 = call-poly <vilib>:"Mean.vi"("X"=w2209) -> ("mean"=w2208:dbl)  [unwired: 1 out]
    n1746 = case shown="True" w2412 {
      tunnel: w2411 -> [w2723 w2730]
      tunnel: [w2723 w2728] -> w2357
      tunnel: w2409 -> [_ w2725]
      tunnel: w2408 -> [_ w2729]
      tunnel: w2296 -> [w2722 w2727]
      tunnel: [w2722 w2724] -> w2293
      frame False {
      }
      frame True {
        n1747 = Subtract(x=w2729, y=w2725) -> (x-y=w2726:dbl)
        n1748 = Array Subset(array=w2730, index=w2726, length=w2725) -> (w2728:u32[])
        n1749 = Array Subset(array=w2727, index=w2726, length=w2725) -> (w2724:u32[])
      }
    }
    n1750 = feedback-in #3(w2357) -> ()
    n1751 = feedback-in #4(w2293) -> ()
    n1752 = Or(x=w2422, y=w2418) -> (x .or. y?=w2419:bool)
    n1753 = Square Root(x=w2208) -> (sqrt(x)=w2207:dbl)
    n1754 = Equal?(x="Tab Control 6", y=T36."High Res Display") -> (x = y?=w2347:bool)
    n1755 = Multiply(x="APD Disp. Scale", y=w2298) -> (x*y=w2307:waveform(dbl)[])
    n1756 = Multiply(x="APD Disp. Downsample", y=w2305) -> (x*y=w2303:dbl)
    n1757 = Multiply(x=10.0, y=w2207) -> (x*y=→"Trap 1 Position RMS (A)":dbl)
    n1758 = Divide(x=w2307, y=w2303) -> (x/y=w2275:waveform(dbl)[])
    n1759 = Index Array(array=w2275, index=0) -> (element=w2285:waveform(dbl))
    n1760 = case "For computing FFTs for display" shown="True" "Compute FFT" {
      tunnel: w2302 -> [_ w3400]
      frame False {
      }
      frame True {
        n1761 = Build Array("FFT 1 Choice 1", "FFT 1 Choice 2", "FFT 2 Choice 1", "FFT 2 Choice 2") -> (w3393:u16[])
        n1762 = Array Size(array=w3400) -> (size(s)=w3399:i32)
        n1763 = feedback-in #6(w3393) -> ()
        n1764 = feedback #6(u16[] [100, 100, 100, 100]) -> (w3394:u16[])
        n1765 = feedback-in #7("# Spectra to Ave.") -> ()
        n1766 = feedback #7("# Spectra to Ave.") -> (w3391:dbl)
        n1767 = Not Equal?(x="# Spectra to Ave.", y=w3391) -> (x != y?=w3390:bool)
        n1768 = Not Equal?(x=w3393, y=w3394) -> (x != y?=w3392:bool)
        n1769 = feedback #8(1.0) -> (w3377:dbl)
        n1770 = Compound Arithmetic op=OR("Reset FFT", w3392, w3390) -> (w3375:bool)
        n1771 = Select(t=1.0, s=w3375, f=w3377) -> (s? t:f=w3379:dbl)
        n1772 = Greater?(x=w3379, y="# Spectra to Ave.") -> (0:w3398:bool)
        n1773 = Increment(x=w3379) -> (x+1=w3378:dbl)
        n1774 = feedback-in #8(w3378) -> ()
        n1775 = local read "DMA Update Period (s)"() -> (w3373:dbl)
        n1776 = Multiply(x="# Spectra to Ave.", y=w3373) -> (x*y=→"Ave. Time (s)":dbl)
        n1777 = Build Array(cluster{"f0":dbl, "df":dbl, "magnitude":dbl[]} {"f0"=0.0, "df"=0.0, "magnitude"=[]} ("PSD")) -> (w3382:cluster{"f0":dbl, "df":dbl, "magnitude":dbl[]}[])
        n1778 = Build Array(w3382, w3382, w3382, w3382) -> (w3384:T47)
        n1779 = feedback #9(w3384) -> (w3389:T47)
        n1780 = for {
          N: 4 -> [_]
          tunnel: w3393 -> [w3422] mode=indexing
          tunnel: w3400 -> [w3423]
          tunnel: w3399 -> [w3425]
          tunnel: w3375 -> [w3418]
          tunnel: w3398 -> [w3417]
          tunnel: "# Spectra to Ave." -> [w3416]
          tunnel: [w3415] -> w3388 mode=indexing
          tunnel: w3389 -> [w3420] mode=indexing
          tunnel: [w3419] -> w3376 mode=indexing
          tunnel: w3379 -> [w3414]
          n1781 = Less?(x=w3422, y=w3425) -> (x < y?=w3424:bool)
          n1782 = Index Array(array=w3423, index=w3422) -> (element=w3421:waveform(dbl))
          n1783 = case shown="True" w3424 {
            tunnel: w3421 -> [_ w3442]
            tunnel: w3420 -> [w3427 w3440]
            tunnel: [w3427 w3428] -> w3419
            tunnel: w3418 -> [_ w3439]
            tunnel: w3417 -> [_ w3432]
            tunnel: w3416 -> [_ w3431]
            tunnel: [cluster{"f0":dbl, "df":dbl, "magnitude":dbl[]} {"f0"=0.0, "df"=0.0, "magnitude"=[]} ("PSD") w3433] -> w3415
            tunnel: w3414 -> [_ w3430]
            frame False {
            }
            frame True {
              n1784 = call <vilib>:"Std Deviation and Variance.vi"("X"=w3442) -> ("mean"=w3443:dbl)  [unwired: 1 in, 2 out]
              n1785 = Subtract(x=w3442, y=w3443) -> (x-y=w3441:waveform(dbl))
              n1786 = xnode "Spectral Measurements"("Signals"=w3441) -> ("PSD"=w3435:cluster{"f0":dbl, "df":dbl, "magnitude":dbl[]})  [unwired: 1 in, 1 out]
              n1787 = case shown="False" w3439 {
                tunnel: w3440 -> [w3452 _]
                tunnel: [w3448 w3457] -> w3428
                tunnel: w3435 -> [w3451 w3458]
                tunnel: w3432 -> [w3450 _]
                frame False {
                  n1788 = Build Array (concatenate)(w3452, w3451) -> (w3449:cluster{"f0":dbl, "df":dbl, "magnitude":dbl[]}[])
                  n1789 = case shown="True" w3450 {
                    tunnel: w3449 -> [w3453 w3456]
                    tunnel: [w3453 w3454] -> w3448
                    frame False {
                    }
                    frame True {
                      n1790 = Delete From Array(array=w3456, index=0) -> (array with subset deleted=w3454:cluster{"f0":dbl, "df":dbl, "magnitude":dbl[]}[])  [unwired: 1 in, 1 out]
                    }
                  }
                }
                frame True {
                  n1791 = Build Array(w3458) -> (w3457:cluster{"f0":dbl, "df":dbl, "magnitude":dbl[]}[])
                }
              }
              n1792 = for {
                tunnel: w3428 -> [w3447] mode=indexing
                tunnel: [w3446] -> w3438 mode=indexing
                workers-P: _ -> [_]
                n1793 = Unbundle By Name(w3447) -> ("magnitude"=w3446:dbl[])
              }
              n1794 = Transpose 2D Array(2D array=w3438) -> (transposed array=w3437:dbl[][])
              n1795 = for {
                tunnel: w3437 -> [w3445] mode=indexing
                tunnel: [w3444] -> w3436 mode=indexing
                workers-P: _ -> [_]
                n1796 = Add Array Elements(numeric array=w3445) -> (sum=w3444:dbl)
              }
              n1797 = Select(t=w3431, s=w3432, f=w3430) -> (s? t:f=w3429:dbl)
              n1798 = Divide(x=w3436, y=w3429) -> (x/y=w3434:dbl[])
              n1799 = Bundle By Name(cluster=w3435, "magnitude"=w3434) -> (w3433:cluster{"f0":dbl, "df":dbl, "magnitude":dbl[]})
            }
          }
        }
        n1800 = case shown="True" w3375 {
          tunnel: w3376 -> [w3407 w3413]
          tunnel: [w3407 w3408] -> w3374
          frame False {
          }
          frame True {
            n1801 = Array Subset(array=w3413, index (row)=0 ("index"), length (row)=4 ("length"), index (col)=0 ("index"), length (col)=1 ("length")) -> (w3408:T47)
          }
        }
        n1802 = feedback-in #9(w3374) -> ()
        n1803 = Split 1D Array(array=w3388, index=2) -> (first subarray=→"FFT 1":cluster{"f0":dbl, "df":dbl, "magnitude":dbl[]}[], second subarray=→"FFT 2":cluster{"f0":dbl, "df":dbl, "magnitude":dbl[]}[])
      }
    }
    n1804 = Index Array(array=w2275, index=1) -> (element=w2283:waveform(dbl))
    n1805 = case "For displaying the high resolution display (no downsampling)" shown="True" w2347 {
      tunnel: w2302 -> [_ w2623]
      frame False {
      }
      frame True {
        n1806 = Index Array(array=w2623, index="High Res. Display") -> (element=w2624:waveform(dbl))
        n1807 = call <vilib>:"Std Deviation and Variance.vi"("X"=w2624) -> ("mean"=w2631:dbl, "standard deviation"=w2636:dbl)  [unwired: 1 in, 1 out]
        "Mean Intensity" <- w2631
        "Sigma" <- w2636
        n1808 = Subtract(x=w2624, y=w2631) -> (x-y=w2630:waveform(dbl))
        n1809 = Select(t=w2630, s="Subtract mean", f=w2624) -> (s? t:f=→"1 Channel":waveform(dbl))
        n1810 = Divide(x=w2636, y=w2631) -> (x/y=→"Sigma/Mean":dbl)
        n1811 = feedback #10(1) -> (w2625:i32)
        n1812 = Greater Or Equal?(x=w2625, y="Slow mean N ave.") -> (x >= y?=w2638:bool)
        n1813 = Increment(x=w2625) -> (x+1=w2640:i32)
        n1814 = Select(t=1, s=w2638, f=w2640) -> (s? t:f=w2627:i32)
        n1815 = feedback-in #10(w2627) -> ()
        n1816 = feedback #11() -> (w2628:waveform(dbl))  [unwired: 1 out]
        n1817 = case shown="Default" w2625 {
          tunnel: [w2643 w2646] -> w2629
          tunnel: w2628 -> [w2645 _]
          tunnel: w2624 -> [w2644 w2646]
          frame Default {
            n1818 = call-poly <vilib>:"Append Waveforms.vi"("waveform B"=w2644, "waveform A"=w2645) -> ("waveform out"=w2643:waveform(dbl))  [unwired: 1 in, 8 out]
          }
          frame 1 {
          }
        }
        n1819 = feedback-in #11(w2629) -> ()
        n1820 = case shown="True" w2638 {
          tunnel: w2629 -> [_ w2642]
          frame False {
          }
          frame True {
            n1821 = call-poly <vilib>:"Mean.vi"("X"=w2642) -> ("mean"=→"Slow mean":dbl)  [unwired: 1 out]
          }
        }
      }
    }
    n1822 = case "For plotting results of scanning MCL" shown="True" w2419 {
      tunnel: w2418 -> [_ w2763]
      tunnel: w2340 -> [_ w2859]
      tunnel: w2427 -> [_ _]
      tunnel: w2302 -> [_ w2833]
      tunnel: w2277 -> [_ w2764]
      tunnel: w2276 -> [_ w2737]
      frame False {
      }
      frame True {
        w2744 = u32 0 items=["Horizontal", "Vertical", "Central", "1st Diagonal", "2nd Diagonal"] ("Type of Symmetry")
        w2772 = u32 0 items=["Horizontal", "Vertical", "Central", "1st Diagonal", "2nd Diagonal"] ("Type of Symmetry")
        w2775 = u32 0 items=["Horizontal", "Vertical", "Central", "1st Diagonal", "2nd Diagonal"] ("Type of Symmetry")
        w2804 = u32 0 items=["Horizontal", "Vertical", "Central", "1st Diagonal", "2nd Diagonal"] ("Type of Symmetry")
        n1823 = Index Array(array=w2833, index=10) -> (element=w2839:waveform(dbl))
        n1824 = Index Array(array=w2833, index=11) -> (element=w2836:waveform(dbl))
        n1825 = local read "Cycles/step (MCL)"() -> (w2789:u64)
        n1826 = Index Array(array=w2833, index="Channel") -> (element=w2835:waveform(dbl))
        n1827 = Unbundle(w2737) -> ("New Image"=w2736:T3, "New Image"=w2735:T3, "New Image"=w2734:T3, "New Image"=w2733:T3)
        n1828 = Unbundle By Name(w2839) -> ("Y"=w2791:dbl[])
        n1829 = Unbundle By Name(w2836) -> ("Y"=w2793:dbl[])
        n1830 = Unbundle By Name(w2835) -> ("Y"=w2798:dbl[])
        n1831 = call "downsample 1D array - double.vi"("Ave N"=w2789, "Array In"=w2791) -> ("Array Out"=w2790:dbl[])  [unwired: 1 out]
        n1832 = call "downsample 1D array - double.vi"("Ave N"=w2789, "Array In"=w2793) -> ("Array Out"=w2792:dbl[])  [unwired: 1 out]
        n1833 = call "downsample 1D array - double.vi"("Ave N"=w2789, "Array In"=w2798) -> ("Array Out"=w2797:dbl[])  [unwired: 1 out]
        n1834 = feedback #12(w2859) -> (w2860:dbl[])
